vi "test Verify Hello VITester.vi"(8 "error in (no error)":errorcluster, 11 "Testing Approval Tests in":refnum<class "VITester Extension Tests.lvclass">) -> (0 "error out":errorcluster, 3 "Testing Approval Tests out":refnum<class "VITester Extension Tests.lvclass">)   [LabVIEW 2020, in "VITester Extension Tests.lvclass"]
uses:
  VITester Extension Tests.lvclass
  C:/Program Files/National Instruments/LabVIEW 2020/vi.lib/addons/_JKI Toolkits/VI Tester/TestCase.llb/TestCase.lvclass
  Extensions/VITester.Extension/VITester.Extension.lvlib
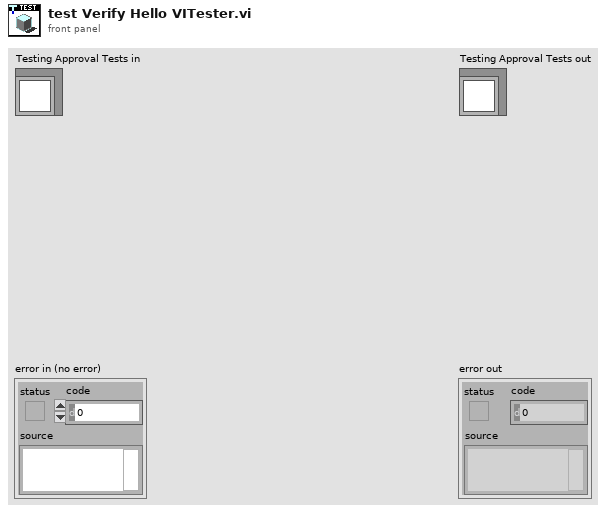
[diagram p1: front panel]
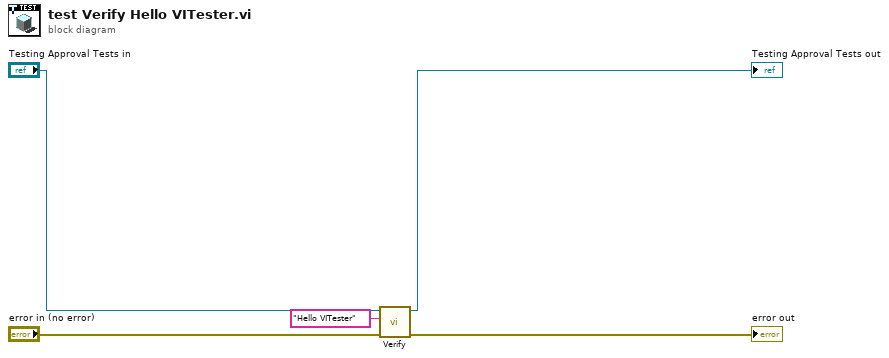
[diagram p0: block diagram]
diagram:
  n1 = call "Verify.vi"("error in"="error in (no error)", "Test Data"="Hello VITester", "TestCase"="Testing Approval Tests in") -> ("error out"=→"error out":errorcluster, "TestCase"=→"Testing Approval Tests out":refnum<class "VITester Extension Tests.lvclass">)  [unwired: 7 in]
